vi "Read Root Lifetime.vi"(7 "Actor in":refnum<class "Actor.lvclass">) -> (2 "Root Lifetime":refnum<data-value>)   [LabVIEW 2020, in "jettl.lvlib"]
uses:
  jettl.lvlib
  Actor/Actor.lvclass
  Msg/Msg.lvclass
  Refs/Refs.lvclass
  Root Lifetime.ctl
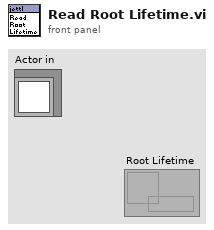
[diagram p1: front panel]
types:
  T1 = typedef "jettl.lvlib/Root Lifetime.ctl" = cluster{"Edge Layers":refnum<class "Actor.lvclass">[], "Core Layers":refnum<class "Actor.lvclass">[]}
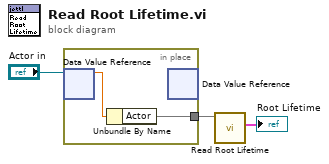
[diagram p0: block diagram]
diagram:
  n1 = in-place {
    in-place-border: [w4] -> w1
    n2 = in-place-dvr #1("Actor in") -> (w5:dbl)  [unwired: 1 out]
    n3 = Unbundle By Name(w5) -> ("Actor"=w4)
    n4 = in-place-dvr #1() -> ()  [unwired: 1 in, 2 out]
  }
  n5 = call-dynamic "Read Root Lifetime.vi"("Actor in"=w1) -> ("Root Lifetime"=→"Root Lifetime":T1)  [unwired: 10 in]
